vi "test_libssh2_sftp_opendir.vi"() -> ()   [LabVIEW 2013, in "libssh2_integration_tests.lvlib"]
uses:
  libssh2_integration_tests.lvlib
  <vilib>/addons/_JKI Toolkits/Caraya/classes/Test/Test.lvclass
  <vilib>/addons/_JKI Toolkits/Caraya/classes/Assert/Assert.lvclass
  libssh2/libssh2.lvlib
panel:
  out "error out":errorcluster
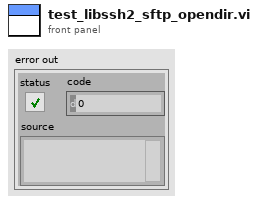
[diagram p1: front panel]
types:
  T1 = typedef "libssh2.lvlib/Session Refnum.ctl" = refnum<k1>
  T2 = typedef "libssh2.lvlib/SFTP Refnum.ctl" = refnum<k1>
  T3 = typedef "libssh2.lvlib/SFTP Handle Refnum.ctl" = refnum<k1>
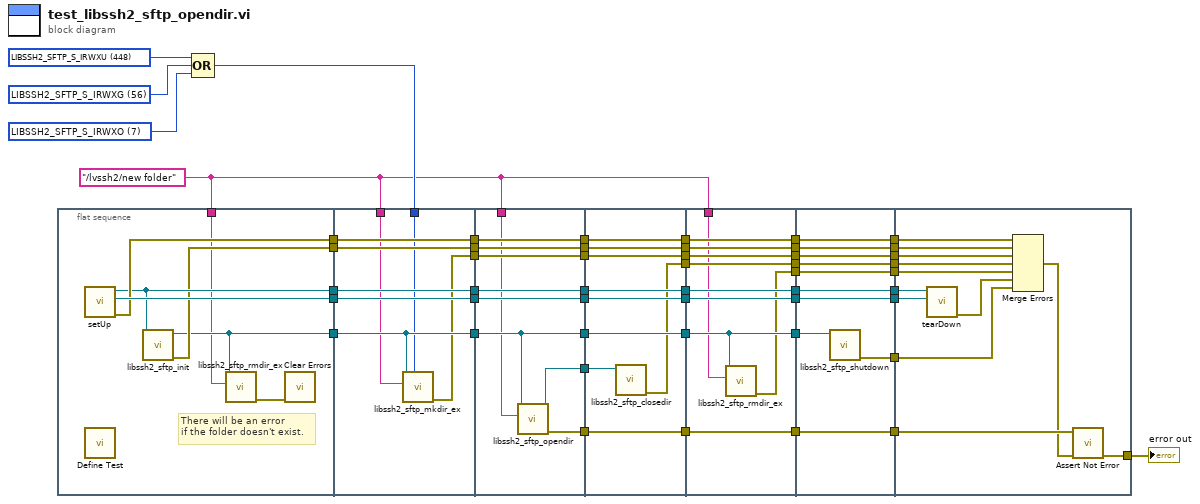
[diagram p0: block diagram]
diagram:
  w3 = "/lvssh2/new folder" ("filename")
  w43 = 7 items=["LIBSSH2_SFTP_S_IRWXU"=448, "LIBSSH2_SFTP_S_IRUSR"=256, "LIBSSH2_SFTP_S_IWUSR"=128, "LIBSSH2_SFTP_S_IXUSR"=64, "LIBSSH2_SFTP_S_IRWXG"=56, "LIBSSH2_SFTP_S_IRGRP"=32, "LIBSSH2_SFTP_S_IWGRP"=16, "LIBSSH2_SFTP_S_IXGRP"=8, "LIBSSH2_SFTP_S_IRWXO"=7, "LIBSSH2_SFTP_S_IROTH"=4, "LIBSSH2_SFTP_S_IWOTH"=2, "LIBSSH2_SFTP_S_IXOTH"=1] ("mode")
  w44 = 56 items=["LIBSSH2_SFTP_S_IRWXU"=448, "LIBSSH2_SFTP_S_IRUSR"=256, "LIBSSH2_SFTP_S_IWUSR"=128, "LIBSSH2_SFTP_S_IXUSR"=64, "LIBSSH2_SFTP_S_IRWXG"=56, "LIBSSH2_SFTP_S_IRGRP"=32, "LIBSSH2_SFTP_S_IWGRP"=16, "LIBSSH2_SFTP_S_IXGRP"=8, "LIBSSH2_SFTP_S_IRWXO"=7, "LIBSSH2_SFTP_S_IROTH"=4, "LIBSSH2_SFTP_S_IWOTH"=2, "LIBSSH2_SFTP_S_IXOTH"=1] ("mode")
  w45 = 448 items=["LIBSSH2_SFTP_S_IRWXU"=448, "LIBSSH2_SFTP_S_IRUSR"=256, "LIBSSH2_SFTP_S_IWUSR"=128, "LIBSSH2_SFTP_S_IXUSR"=64, "LIBSSH2_SFTP_S_IRWXG"=56, "LIBSSH2_SFTP_S_IRGRP"=32, "LIBSSH2_SFTP_S_IWGRP"=16, "LIBSSH2_SFTP_S_IXGRP"=8, "LIBSSH2_SFTP_S_IRWXO"=7, "LIBSSH2_SFTP_S_IROTH"=4, "LIBSSH2_SFTP_S_IWOTH"=2, "LIBSSH2_SFTP_S_IXOTH"=1] ("mode")
  n1 = flat-sequence {
    tunnel: [w56] -> w51
    tunnel: [w58] -> w50
    tunnel: [w57] -> w49
    tunnel: [w55] -> w47
    tunnel: [w54] -> w46
    tunnel: w3 -> [w53]
    tunnel: w51 -> [w66]
    tunnel: w50 -> [w65]
    tunnel: [w66] -> w34
    tunnel: [w65] -> w33
    tunnel: [w62] -> w32
    tunnel: [w64] -> w31
    tunnel: w49 -> [w64]
    tunnel: w47 -> [w63]
    tunnel: [w63] -> w30
    tunnel: w46 -> [w62]
    tunnel: w42 -> [w61]
    tunnel: w3 -> [w60]
    tunnel: [w59] -> w29
    tunnel: w34 -> [w75]
    tunnel: [w75] -> w28
    tunnel: w33 -> [w74]
    tunnel: [w74] -> w27
    tunnel: w32 -> [w69]
    tunnel: [w69] -> w26
    tunnel: w31 -> [w73]
    tunnel: [w73] -> w25
    tunnel: w30 -> [w72]
    tunnel: [w72] -> w24
    tunnel: w29 -> [w71]
    tunnel: [w71] -> w23
    tunnel: [w70] -> w22
    tunnel: w3 -> [w68]
    tunnel: [w67] -> w21
    tunnel: w28 -> [w84]
    tunnel: [w84] -> w19
    tunnel: w27 -> [w83]
    tunnel: [w83] -> w17
    tunnel: w26 -> [w82]
    tunnel: [w82] -> w15
    tunnel: w25 -> [w81]
    tunnel: [w81] -> w13
    tunnel: w24 -> [w80]
    tunnel: [w80] -> w11
    tunnel: w23 -> [w79]
    tunnel: [w79] -> w9
    tunnel: w22 -> [w78]
    tunnel: [w78] -> w7
    tunnel: w21 -> [w77]
    tunnel: [w76] -> w5
    tunnel: w19 -> [w94]
    tunnel: [w94] -> w18
    tunnel: w17 -> [w93]
    tunnel: [w93] -> w16
    tunnel: w15 -> [w87]
    tunnel: [w87] -> w14
    tunnel: w13 -> [w92]
    tunnel: [w92] -> w12
    tunnel: w11 -> [w91]
    tunnel: [w91] -> w10
    tunnel: w9 -> [w90]
    tunnel: [w90] -> w8
    tunnel: w7 -> [w89]
    tunnel: [w89] -> w6
    tunnel: w5 -> [w88]
    tunnel: [w88] -> w4
    tunnel: w3 -> [w86]
    tunnel: [w85] -> w2
    tunnel: w18 -> [w104]
    tunnel: [w104] -> w41
    tunnel: w16 -> [w103]
    tunnel: [w103] -> w40
    tunnel: w14 -> [w100]
    tunnel: [w97] -> w39
    tunnel: w12 -> [w102]
    tunnel: [w102] -> w38
    tunnel: w10 -> [w101]
    tunnel: [w101] -> w37
    tunnel: [w99] -> w36
    tunnel: w8 -> [w98]
    tunnel: [w98] -> w35
    tunnel: w6 -> [w97]
    tunnel: w4 -> [w96]
    tunnel: [w96] -> w20
    tunnel: w2 -> [w95]
    tunnel: [w95] -> w1
    tunnel: w41 -> [w116]
    tunnel: w40 -> [w115]
    tunnel: w39 -> [w114]
    tunnel: w38 -> [w113]
    tunnel: [w110] -> w48
    tunnel: w37 -> [w109]
    tunnel: w36 -> [w108]
    tunnel: w35 -> [w107]
    tunnel: w20 -> [w106]
    tunnel: w1 -> [w105]
    frame #0 {
      # "There will be an error\nif the folder doesn't exist."
      n2 = call "setUp.vi"() -> ("error out"=w57:errorcluster, "connection ID"=w58:refnum<k5>, "session"=w56:T1)  [unwired: 9 in]
      n3 = call <vilib>:"Define Test.vi"() -> ()  [unwired: 10 in, 2 out]
      n4 = call "libssh2_sftp_init.vi"("session"=w56) -> ("error out"=w55:errorcluster, "sftp"=w54:T2)  [unwired: 9 in]
      n5 = call "libssh2_sftp_rmdir_ex.vi"("path"=w53, "sftp"=w54) -> ("error out"=w52:errorcluster)  [unwired: 9 in]
      n6 = call <vilib>:"Clear Errors.vi"("error in (no error)"=w52) -> ()  [unwired: 6 in, 1 out]
    }
    frame #1 {
      n7 = call "libssh2_sftp_mkdir_ex.vi"("mode"=w61, "path"=w60, "sftp"=w62) -> ("error out"=w59:errorcluster)  [unwired: 8 in]
    }
    frame #2 {
      n8 = call "libssh2_sftp_opendir.vi"("path"=w68, "sftp"=w69) -> ("error out"=w70:errorcluster, "sftp handle"=w67:T3)  [unwired: 8 in]
    }
    frame #3 {
      n9 = call "libssh2_sftp_closedir.vi"("sftp handle"=w77) -> ("error out"=w76:errorcluster)  [unwired: 10 in]
    }
    frame #4 {
      n10 = call "libssh2_sftp_rmdir_ex.vi"("path"=w86, "sftp"=w87) -> ("error out"=w85:errorcluster)  [unwired: 9 in]
    }
    frame #5 {
      n11 = call "libssh2_sftp_shutdown.vi"("sftp"=w100) -> ("error out"=w99:errorcluster)  [unwired: 10 in]
    }
    frame #6 {
      n12 = call "tearDown.vi"("connection ID"=w115, "session"=w116) -> ("error out"=w112:errorcluster)  [unwired: 9 in]
      n13 = Merge Errors(w113, w109, w107, w106, w105, w112, w108) -> (w111:errorcluster)
      n14 = call <vilib>:"Assert Not Error.vi"("error in (no error)"=w111, "Not Error?"=w114) -> ("error out"=w110:errorcluster)  [unwired: 8 in, 1 out]
    }
  }
  n15 = Compound Arithmetic op=OR(w45, w44, w43) -> (w42:i32)
  "error out" <- w48
